vi "angle_to_position.vi"(10 "arm length":dbl, 11 "angle":dbl) -> (2 "y position":dbl, 3 "x position":dbl)   [LabVIEW 2017]
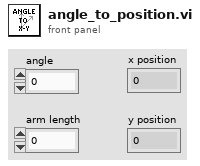
[diagram p1: front panel]
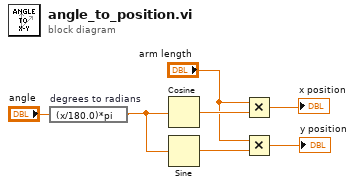
[diagram p0: block diagram]
diagram:
  n1 = expression code="(x/180.0)*pi" "degrees to radians"("angle") -> (w2:dbl)
  n2 = Cosine(x=w2) -> (cos(x)=w7:dbl)
  n3 = Sine(x=w2) -> (sin(x)=w6:dbl)
  n4 = Multiply(x="arm length", y=w7) -> (x*y=→"x position":dbl)
  n5 = Multiply(x="arm length", y=w6) -> (x*y=→"y position":dbl)
